vi "EventStructureAppExample.vi"() -> ()   [LabVIEW 2019]
panel:
  in  "stop":bool
  out "Boiler":bool
  in  "Temperature":dbl(knob) scale=0.0..100.0
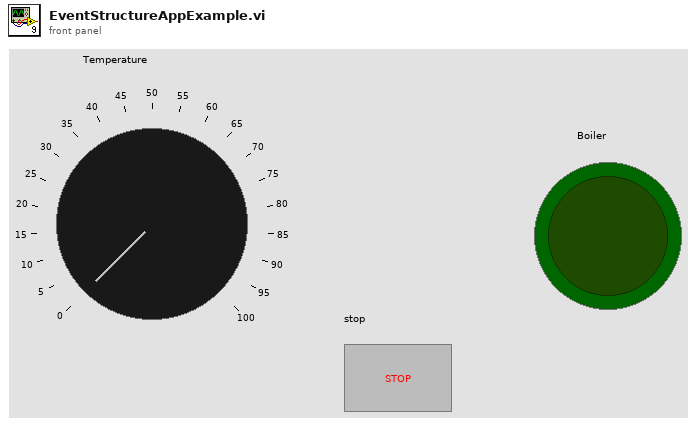
[diagram p1: front panel]
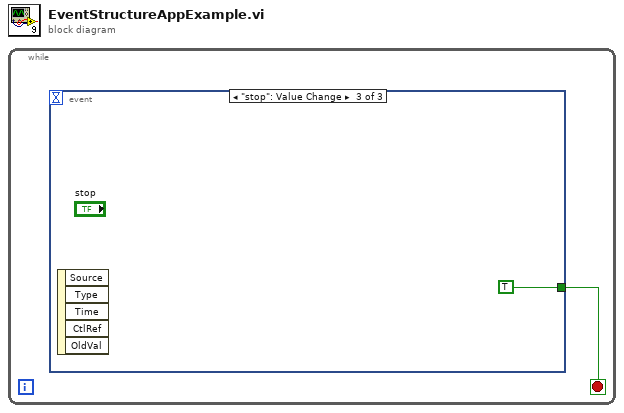
[diagram p0: block diagram]
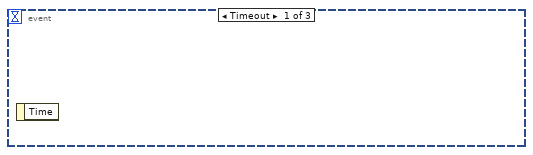
[diagram p2: hidden frame]
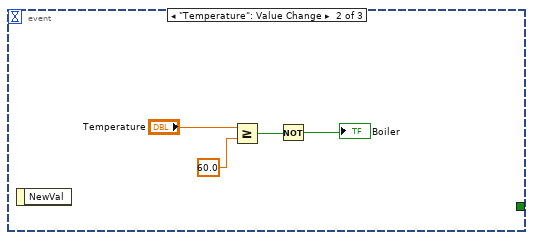
[diagram p3: hidden frame]
diagram:
  n1 = while {
    stop <- w1 stop-if-true
    n2 = event shown="[2] \"stop\": Value Change" {
      selector: _ -> [_ _ _]
      dyn-events: _ -> [_ _ _]
      timeout: _ -> [_ _ _]
      tunnel: [_ _ TRUE] -> w1
      event Timeout {
        n3 = event-data() -> ()  [unwired: 1 in, 1 out]
      }
      event "Temperature": Value Change {
        n4 = event-data() -> ()  [unwired: 1 in, 1 out]
        n5 = Greater Or Equal?(x="Temperature", y=60.0) -> (x >= y?=w4:bool)
        n6 = Not(x=w4) -> (.not. x?=→"Boiler":bool)
      }
      event "stop": Value Change {
        n7 = event-data() -> ()  [unwired: 1 in, 5 out]
      }
    }
  }
